vi "Read Packet.vi"(1 "MSG 2":T1, 2 "MSG 1":T1, 3 "Command":u16(ring) items=["제품명 읽기", "S/N 읽기", "Firmware Version 읽기", "제품 ID 설정", "제품 ID 읽기", "통신 속도 설정", "통신 속도 읽기", "필터 종류 설정", "필터 종류 읽기", "F/T 현재값 출력", "F/T 연속 출력", "F/T 출력 멈춤", "Reserved", "Reserved", "출력 주기 설정", "출력 주기 읽기", "Bias 설정", "Overload log 읽기"]) -> (0 "Response-Packet":string)   [LabVIEW 2011]
panel:
  out "제품명":string
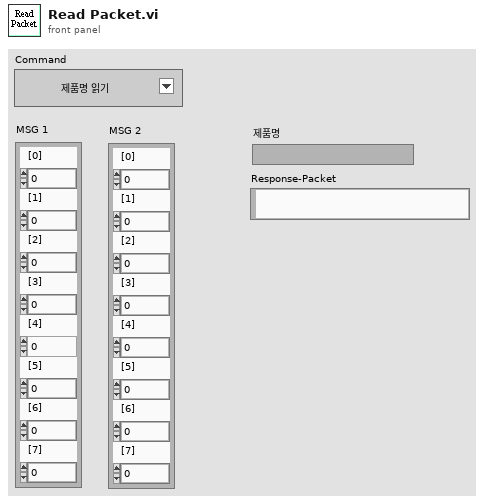
[diagram p1: front panel]
types:
  T1 = cluster{"[0]":u8, "[1]":u8, "[2]":u8, "[3]":u8, "[4]":u8, "[5]":u8, "[6]":u8, "[7]":u8}
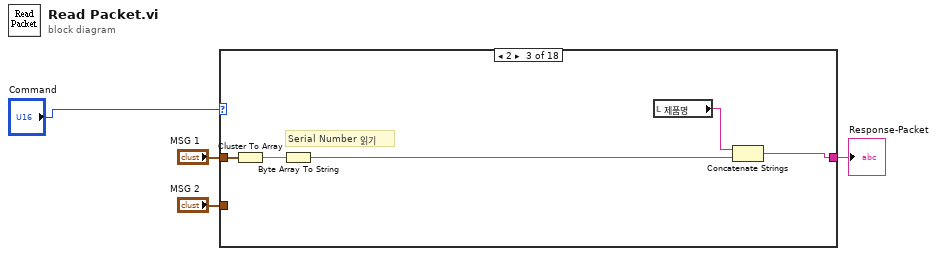
[diagram p0: block diagram]
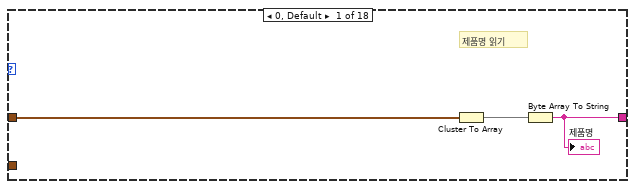
[diagram p2: hidden frame]
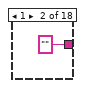
[diagram p3: hidden frame]
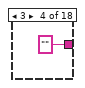
[diagram p4: hidden frame]
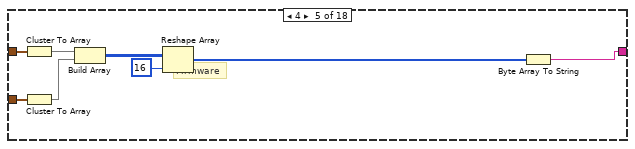
[diagram p5: hidden frame]
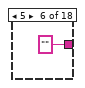
[diagram p6: hidden frame]
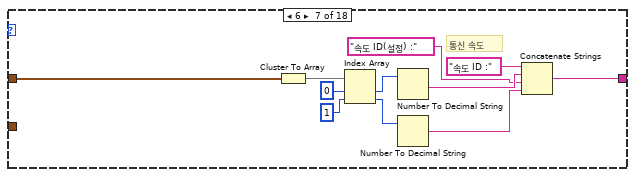
[diagram p7: hidden frame]
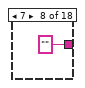
[diagram p8: hidden frame]
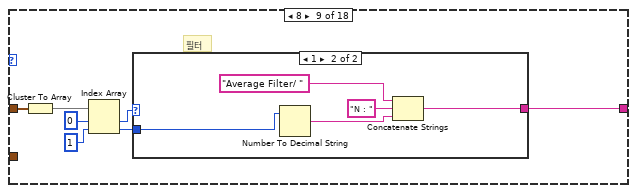
[diagram p9: hidden frame]
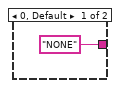
[diagram p10: hidden frame]
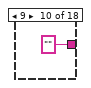
[diagram p11: hidden frame]
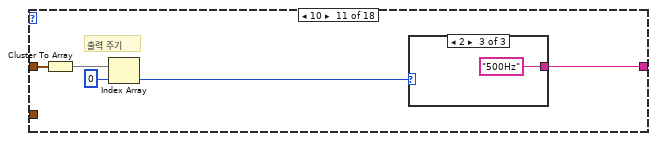
[diagram p12: hidden frame]
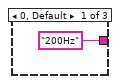
[diagram p13: hidden frame]
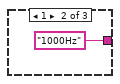
[diagram p14: hidden frame]
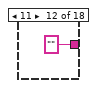
[diagram p15: hidden frame]
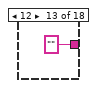
[diagram p16: hidden frame]
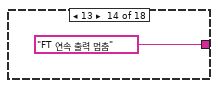
[diagram p17: hidden frame]
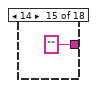
[diagram p18: hidden frame]
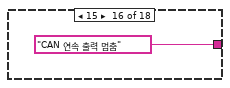
[diagram p19: hidden frame]
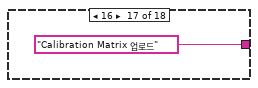
[diagram p20: hidden frame]
diagram:
  n1 = case shown="2" "Command" {
    tunnel: "MSG 1" -> [w7 _ w13 _ w20 _ w34 _ w42 _ w54 _ _ _ _ _ _ _]
    tunnel: "MSG 2" -> [_ _ _ _ w19 _ _ _ _ _ _ _ _ _ _ _ _ _]
    tunnel: [w5 "" ("string") w9 "" ("string") w15 "" ("string") w24 "" ("string") w37 "" ("string") w50 "" ("string") "" ("string") "FT 연속 출력 멈춤" ("string") "" ("string") "CAN 연속 출력 멈춤" ("string") "Calibration Matrix 업로드" ("string") "" ("string")] -> w2
    frame 0, Default {
      # "제품명 읽기"
      n2 = Cluster To Array(cluster=w7) -> (array=w6:u8[])
      n3 = Byte Array To String(unsigned byte array=w6) -> (string=w5:string)
      "제품명" <- w5
    }
    frame 1 {
    }
    frame 2 {
      # "Serial Number 읽기"
      n4 = Cluster To Array(cluster=w13) -> (array=w12:u8[])
      n5 = Byte Array To String(unsigned byte array=w12) -> (string=w11:string)
      n6 = local read "제품명"() -> (w10:string)
      n7 = Concatenate Strings(w10, w11) -> (w9:string)
    }
    frame 3 {
    }
    frame 4 {
      # "Firmware"
      n8 = Cluster To Array(cluster=w20) -> (array=w18:u8[])
      n9 = Cluster To Array(cluster=w19) -> (array=w17:u8[])
      n10 = Build Array(w18, w17) -> (w21:u8[][])
      n11 = Reshape Array(w21, 16 ("차원 크기")) -> (w16:u8[])
      n12 = Byte Array To String(unsigned byte array=w16) -> (string=w15:string)
    }
    frame 5 {
    }
    frame 6 {
      # "통신 속도"
      n13 = Cluster To Array(cluster=w34) -> (array=w33:u8[])
      n14 = Index Array(array=w33, index #1=0 ("인덱스"), index #2=1 ("인덱스")) -> (element #1=w30:u8, element #2=w29:u8)
      n15 = Number To Decimal String(number=w30) -> (decimal integer string=w27:string)  [unwired: 1 in]
      n16 = Number To Decimal String(number=w29) -> (decimal integer string=w25:string)  [unwired: 1 in]
      n17 = Concatenate Strings("속도 ID :" ("문자열"), w27, "속도 ID(설정) :" ("문자열"), w25) -> (w24:string)
    }
    frame 7 {
    }
    frame 8 {
      # "필터"
      n18 = Cluster To Array(cluster=w42) -> (array=w41:u8[])
      n19 = Index Array(array=w41, index #1=0 ("인덱스"), index #2=1 ("인덱스")) -> (element #1=w38:u8, element #2=w36:u8)
      n20 = case shown="1" w38 {
        tunnel: ["NONE" ("string") w44] -> w37
        tunnel: w36 -> [_ w46]
        frame 0, Default {
        }
        frame 1 {
          n21 = Number To Decimal String(number=w46) -> (decimal integer string=w45:string)  [unwired: 1 in]
          n22 = Concatenate Strings("Average Filter/ " ("string"), "N : " ("string"), w45) -> (w44:string)
        }
      }
    }
    frame 9 {
    }
    frame 10 {
      # "출력 주기"
      n23 = Cluster To Array(cluster=w54) -> (array=w53:u8[])
      n24 = Index Array(array=w53, index=0 ("인덱스")) -> (element=w51:u8)
      n25 = case shown="2" w51 {
        tunnel: ["200Hz" ("string") "1000Hz" ("string") "500Hz" ("string")] -> w50
        frame 0, Default {
        }
        frame 1 {
        }
        frame 2 {
        }
      }
    }
    frame 11 {
    }
    frame 12 {
    }
    frame 13 {
    }
    frame 14 {
    }
    frame 15 {
    }
    frame 16 {
    }
    frame 17 {
    }
  }
  "Response-Packet" <- w2
